vi "Turn to Angle.vi"(0 "Current Angle (radians; 0 = right)":dbl, 1 "Target angle":dbl, 2 "Angle Tolerance":dbl=2.0, 3 "PID Gains":T1={"proportional gain (Kc)"=0.6, "integral time (Ti, min)"=0.0, "derivative time (Td, min)"=0.0} {"derivative time (Td, min)" format="%.3f"; "integral time (Ti, min)" format="%.3f"; "proportional gain (Kc)" format="%.3f"}, 4 "Max Output":dbl, 8 "reinitialize? (F)":bool) -> (5 "Turn Speed (subtract from the left motor output)":dbl, 7 "Finished?":bool)   [LabVIEW 2015]
uses:
  <vilib>/addons/control/pid/pid.llb/PID Control Input Filter (DBL).vi
  <vilib>/addons/control/pid/pid.llb/PID (DBL).vi
  <vilib>/addons/control/pid/NI_PID_pid.lvlib
  Team900SwerveDrive/Team900SwerveDrive.lvlib
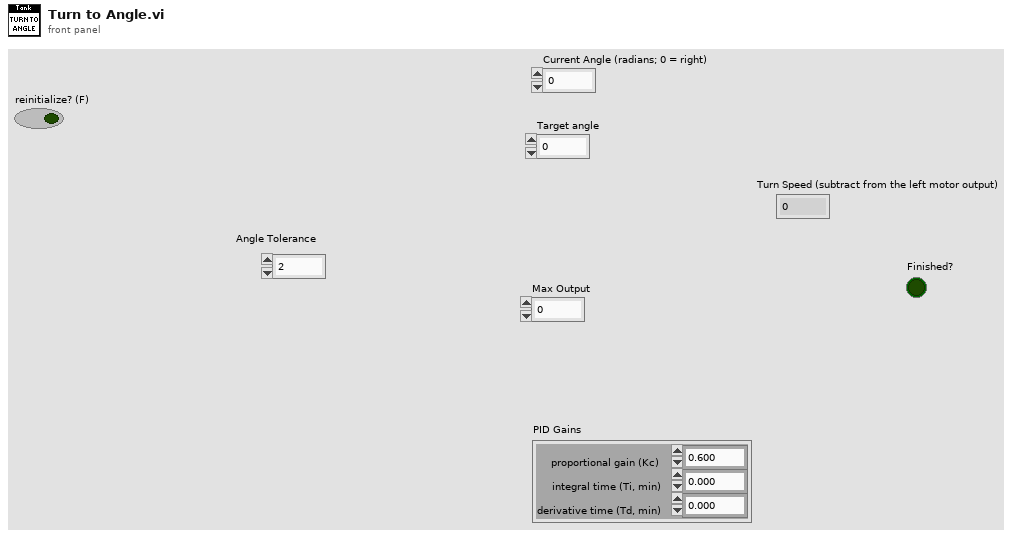
[diagram p1: front panel]
types:
  T1 = cluster{"proportional gain (Kc)":dbl, "integral time (Ti, min)":dbl, "derivative time (Td, min)":dbl}
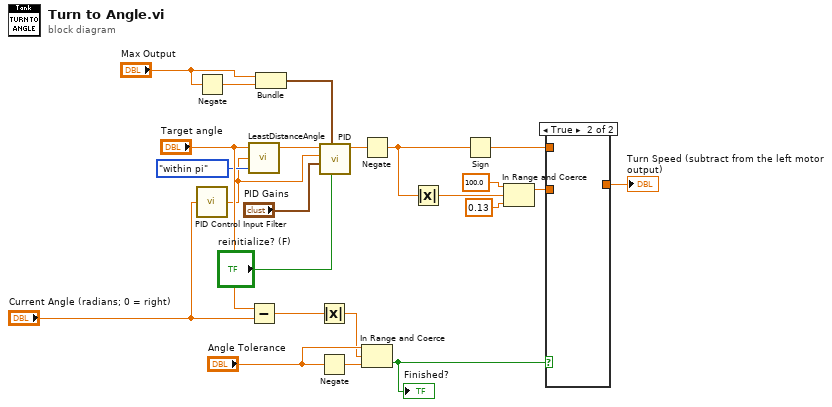
[diagram p0: block diagram]
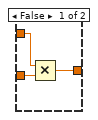
[diagram p2: hidden frame]
diagram:
  n1 = Negate(x="Max Output") -> (-x=w15:dbl)
  n2 = call-poly <vilib>:"PID Control Input Filter.vi"("input"="Current Angle (radians; 0 = right)") -> ("output"=w9:dbl)  [unwired: 4 in]
  n3 = call "LeastDistanceAngle.vi"("Enum"=enum16{"within pi", "within pi/2"}."within pi", "Current angle"=w9, "target angle (between pi and -pi) 2"="Target angle") -> ("output angle"=w10:dbl)  [unwired: 2 out]
  n4 = Subtract(x="Target angle", y="Current Angle (radians; 0 = right)") -> (x-y=w23:dbl)
  n5 = Bundle("Max Output"="Max Output", w15) -> (w14:cluster{"Max Output":dbl, dbl})  [unwired: 1 in]
  n6 = Absolute Value(x=w23) -> (abs(x)=w20:dbl)
  n7 = Negate(x="Angle Tolerance") -> (-x=w21:dbl)
  n8 = call-poly <vilib>:"PID.vi"("reinitialize? (F)"="reinitialize? (F)", "output range"=w14, "PID gains"="PID Gains", "process variable"=w9, "setpoint"=w10) -> ("output"=w17:dbl)  [unwired: 5 in, 1 out]
  n9 = Negate(x=w17) -> (-x=w4:dbl)
  n10 = In Range and Coerce(upper limit="Angle Tolerance", x=w20, lower limit=w21) -> (In Range?=w1:bool)  [unwired: 1 out]
  "Finished?" <- w1
  n11 = Absolute Value(x=w4) -> (abs(x)=w8:dbl)
  n12 = Sign(1:w4) -> (0:w3:dbl)
  n13 = In Range and Coerce(upper limit=100.0, x=w8, lower limit=0.13) -> (coerced(x)=w5:dbl)  [unwired: 1 out]
  n14 = case shown="True" w1 {
    tunnel: w5 -> [w26 _]
    tunnel: w3 -> [w25 _]
    tunnel: [w24 _] -> w2
    frame False {
      n15 = Multiply(x=w25, y=w26) -> (x*y=w24:dbl)
    }
    frame True {
    }
  }
  "Turn Speed (subtract from the left motor output)" <- w2
